vi "log_loop.vi"(8 "error in (no error)":errorcluster, 10 "Log queue":refnum<queue>, 11 "Message Queues":T4) -> (0 "error out":errorcluster)   [LabVIEW 2013]
doc: "Message loop for handling messages pertaining to the acquisition of data from the hardware."
uses:
  queues/que_all_message_queues.ctl
  queues/que_message_cluster.ctl
  gui/type_def/general_and_device.ctl
  gui/type_def/general.ctl
  gui/type_def/device.ctl
  log_state.ctl
  queues/que_enqueue_message_single.vi
  <vilib>/Utility/error.llb/Error Cluster From Error Code.vi
  <vilib>/ErrorRing/Error Ring.xnode
panel:
  out "gral_&_device":T1={"general"={"file_ext"="0.0.0.0", "TCP port"=0, "#devices"=0, "log?"=FALSE, "tcp?"=FALSE, "language"="ENG"}, "eeg_device"={"name"="", "hardware"="", "image"="", "path"=path "", "extra"="", "channels"=""}}
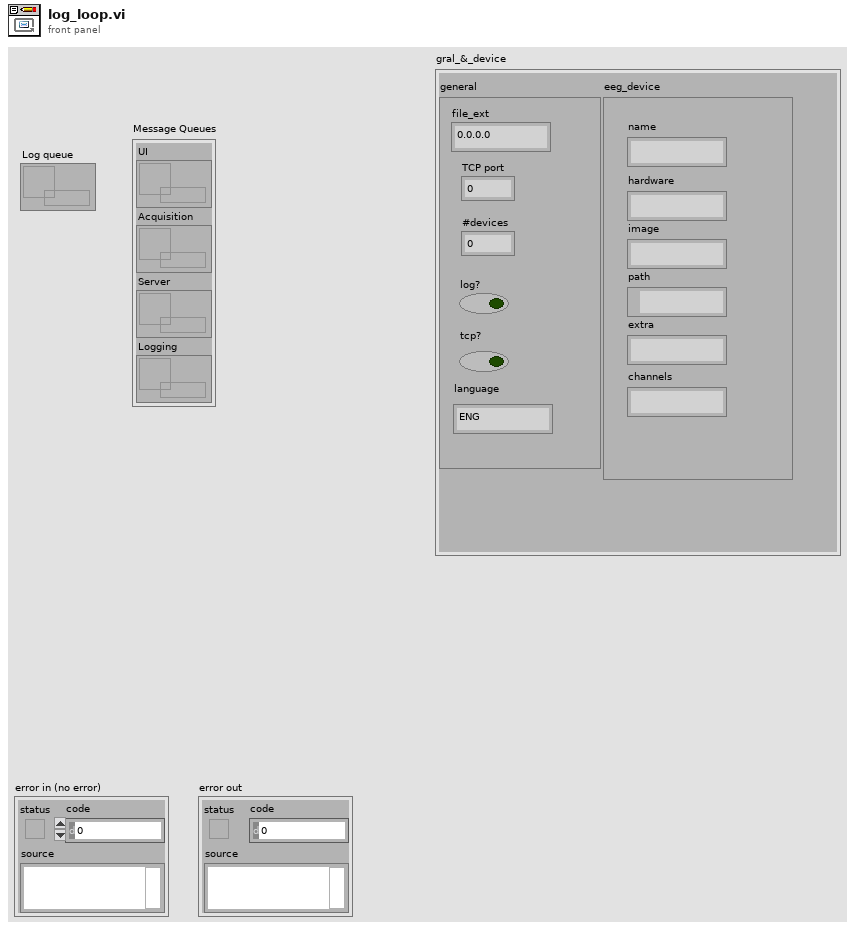
[diagram p1: front panel]
types:
  T1 = typedef "general_and_device.ctl" = cluster{"general":T2, "eeg_device":T3}
  T2 = typedef "general.ctl" = cluster{"file_ext":string, "TCP port":i32, "#devices":i32, "log?":bool, "tcp?":bool, "language":string}
  T3 = typedef "device.ctl" = cluster{"name":string, "hardware":string, "image":string, "path":path, "extra":string, "channels":string}
  T4 = typedef "que_all_message_queues.ctl" = cluster{"UI":refnum<queue>, "Acquisition":refnum<queue>, "Server":refnum<queue>, "Logging":refnum<queue>}
  T5 = typedef "log_state.ctl" = enum16{"Idle", "Logging"}
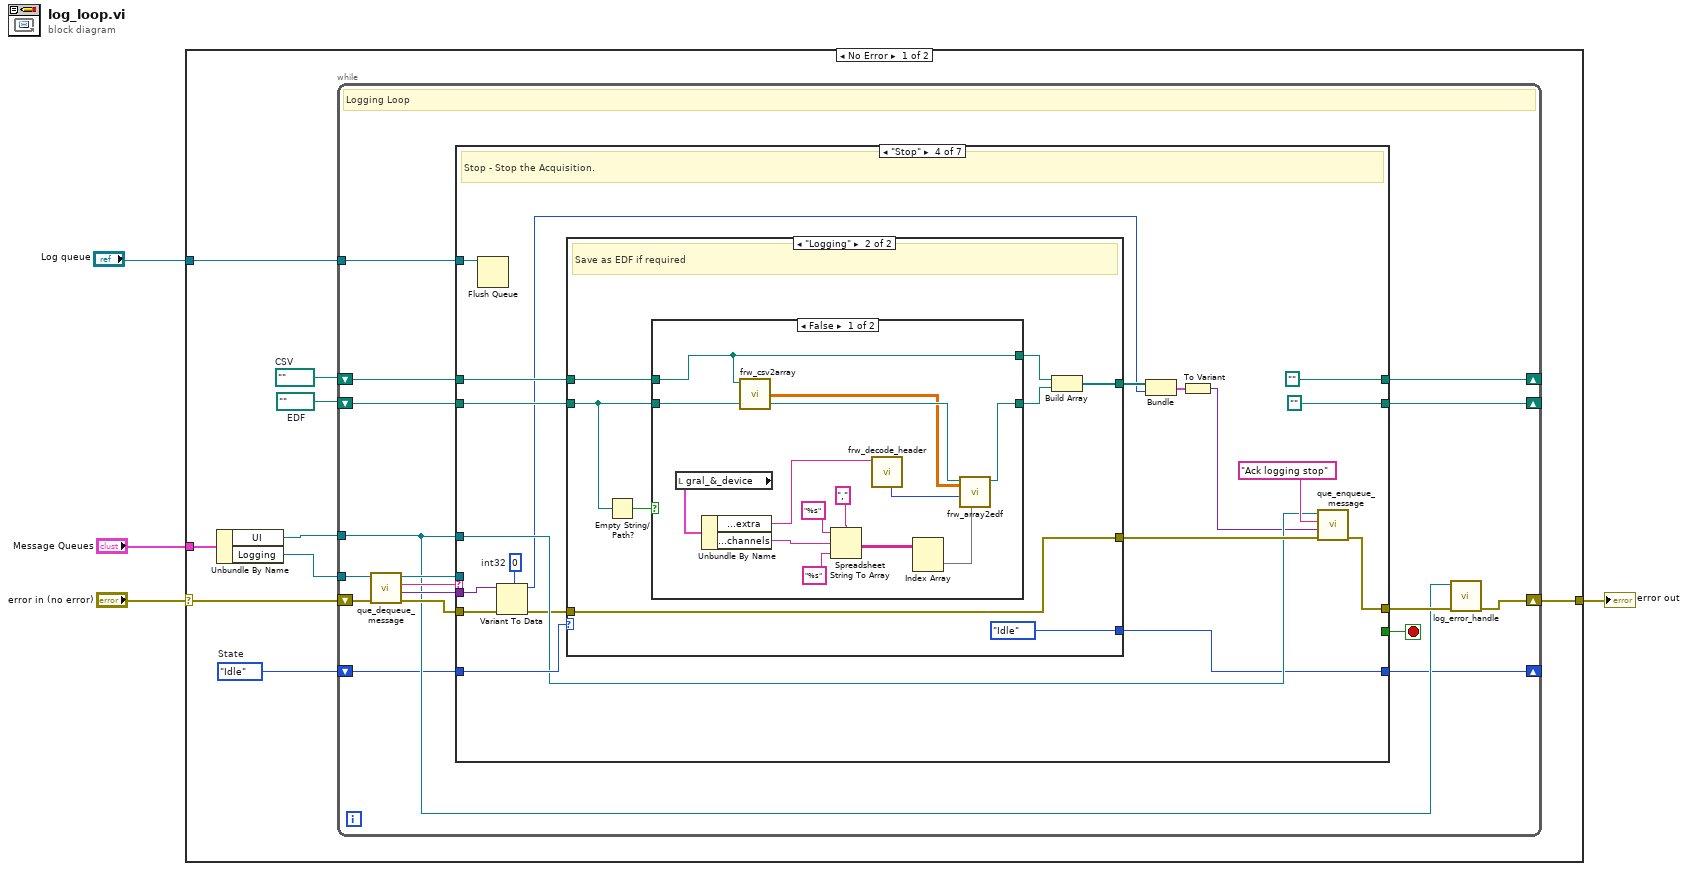
[diagram p0: block diagram]
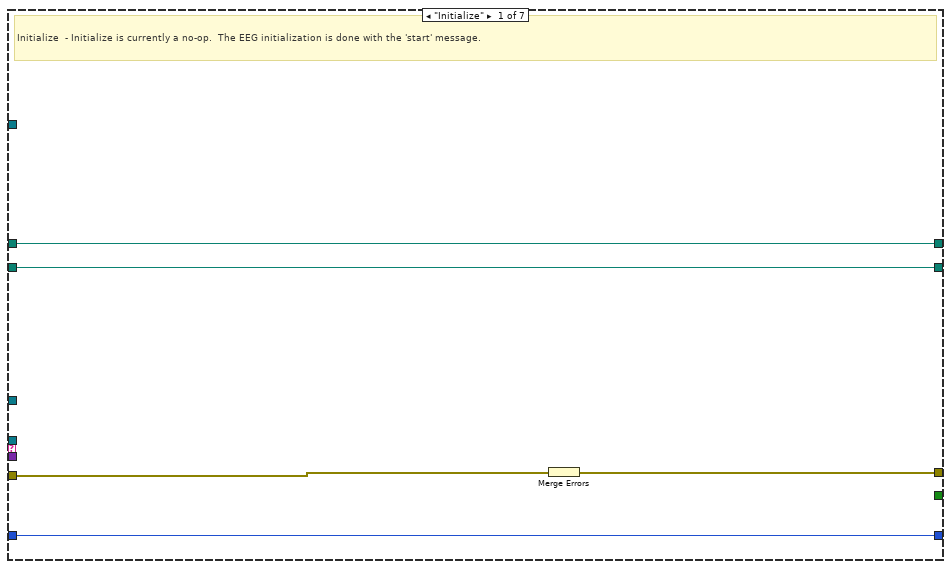
[diagram p2: hidden frame]
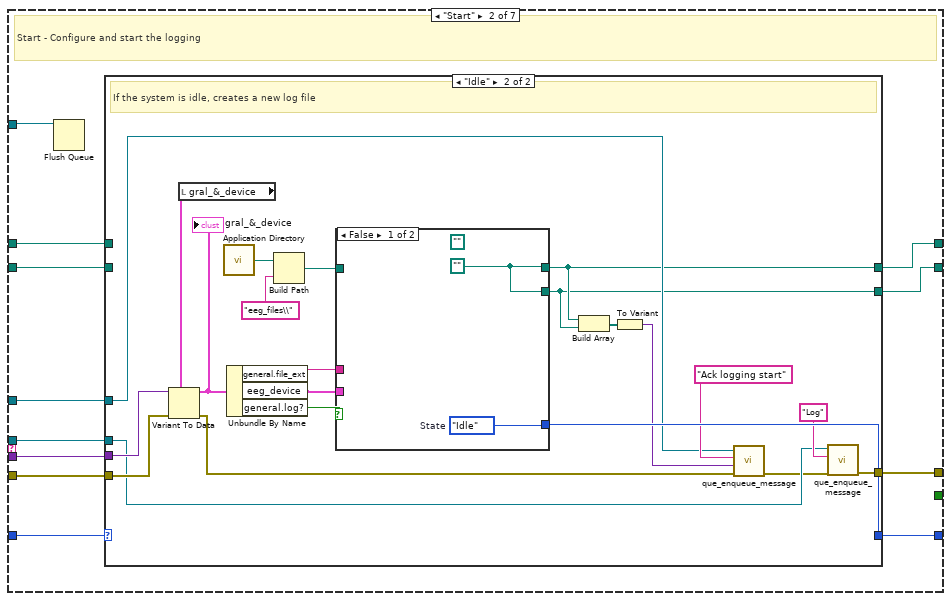
[diagram p3: hidden frame]
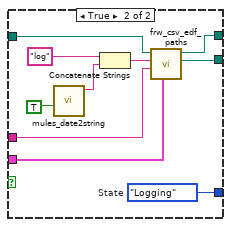
[diagram p5: hidden frame]
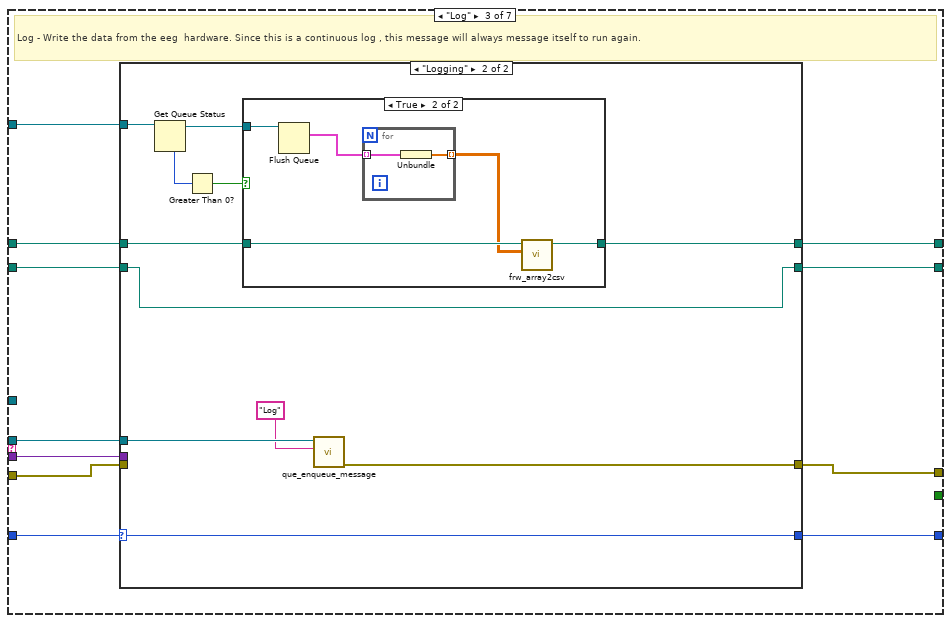
[diagram p6: hidden frame]
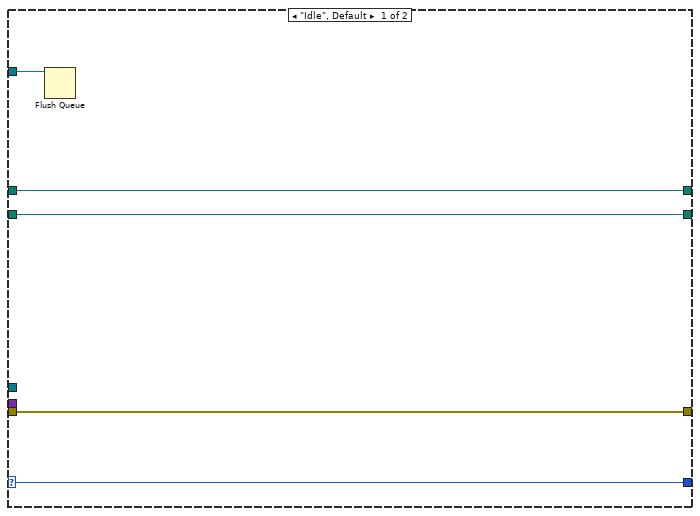
[diagram p7: hidden frame]
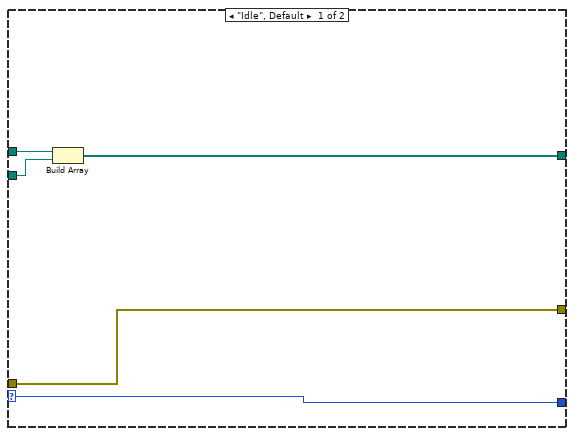
[diagram p9: hidden frame]
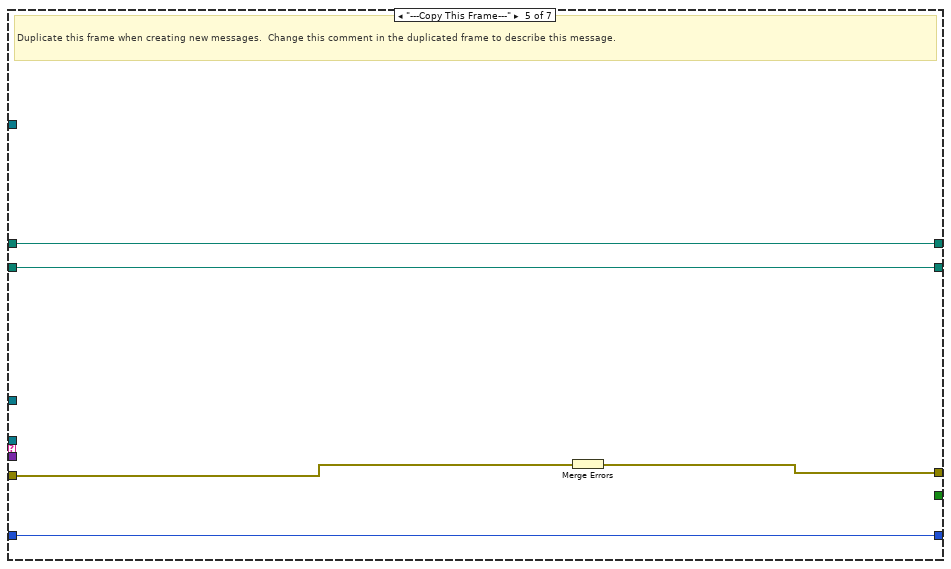
[diagram p11: hidden frame]
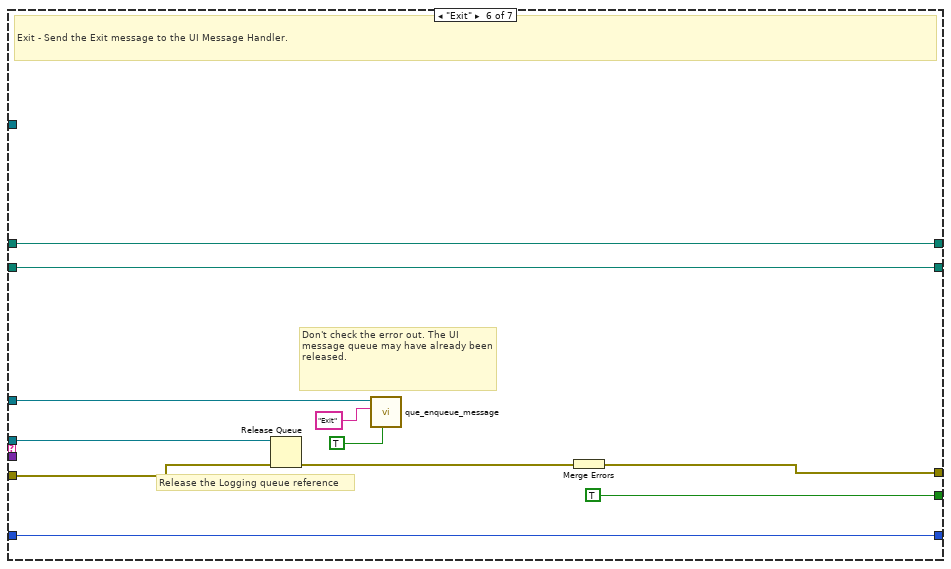
[diagram p12: hidden frame]
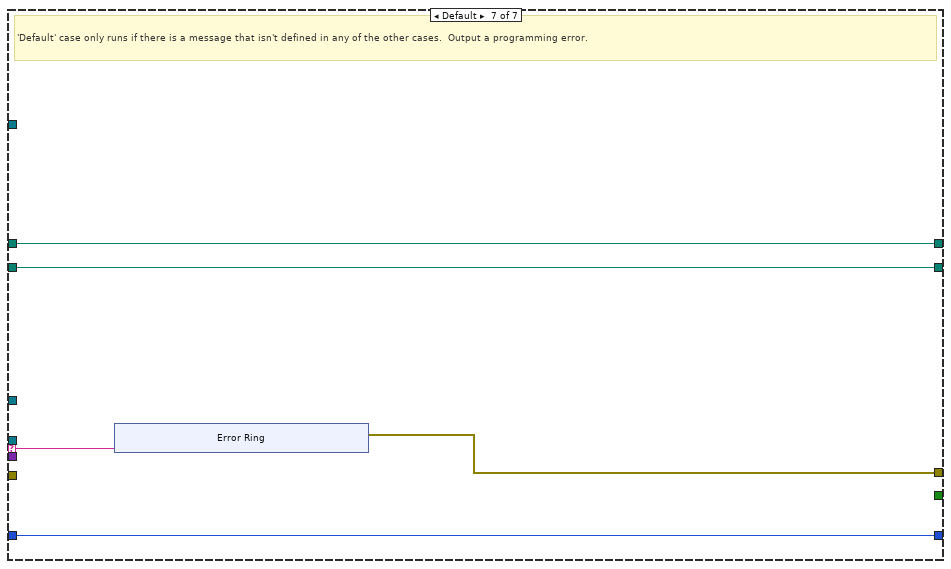
[diagram p13: hidden frame]
diagram:
  n1 = case shown="No Error" "error in (no error)" {
    selector: "error in (no error)" -> [w10 w196]
    tunnel: "Message Queues" -> [w13 _]
    tunnel: [w11 w196] -> w3
    tunnel: "Log queue" -> [w8 _]
    frame No Error {
      w5 = path ""  # EDF
      w7 = path ""  # CSV
      w6 = log_state."Idle"  # State
      n2 = Unbundle By Name(w13) -> ("UI"=w9:refnum<queue>, "Logging"=w12:refnum<queue>)
      n3 = while {
        tunnel: w12 -> [w25]
        shift-right: [w24] -> w11
        shift-left: w10 -> [w29]
        tunnel: w9 -> [w21]
        shift-right: [w20] -> _
        shift-left: w7 -> [w19]
        tunnel: w8 -> [w18]
        shift-right: [w16] -> _
        shift-left: w6 -> [w17]
        shift-right: [w14] -> _
        shift-left: w5 -> [w15]
        stop <- w30 stop-if-true
        # "Logging Loop"
        n4 = call "que_dequeue_message.vi"("error in (no error)"=w29, "Message Queue"=w25) -> ("error out"=w28:errorcluster, "Message Data"=w26:variant, "Message"=w27:string, "dup Message Queue"=w22:refnum<queue>)  [unwired: 6 in]
        n5 = case "Message Cases" shown="\"Stop\"" w27 {
          selector: w27 -> [_ _ _ _ _ _ w186]
          tunnel: w22 -> [_ w47 w95 _ _ w176 _]
          tunnel: w28 -> [w34 w40 w94 w127 w172 w180 _]
          tunnel: [w35 w37 w96 w133 w171 w182 w187] -> w23
          tunnel: [_ _ _ _ _ TRUE _] -> w30
          tunnel: w26 -> [_ w44 w91 w126 _ _ _]
          tunnel: w21 -> [_ w41 _ w135 _ w181 _]
          tunnel: w17 -> [w33 w45 w92 w138 w170 w175 w188]
          tunnel: [w33 w46 w93 w134 w170 w175 w188] -> w16
          tunnel: [w32 w43 w87 path "" w169 w174 w185] -> w20
          tunnel: w19 -> [w32 w42 w90 w137 w169 w174 w185]
          tunnel: w18 -> [_ w36 w89 w121 _ _ _]
          tunnel: w15 -> [w31 w39 w88 w130 w168 w173 w184]
          tunnel: [w31 w38 w86 path "" w168 w173 w184] -> w14
          frame "Initialize" {
            # "Initialize  - Initialize is currently a no-op.  The EEG initialization is done with the 'start' message."
            n6 = Merge Errors(w34) -> (w35:errorcluster)
          }
          frame "Start" {
            # "Start - Configure and start the logging"
            n7 = Flush Queue(queue=w36) -> ()  [unwired: 1 in, 3 out]
            n8 = case shown="\"Idle\"" w45 {
              selector: w45 -> [w50 _]
              tunnel: [w51 w64] -> w37
              tunnel: w40 -> [w51 w72]
              tunnel: w47 -> [_ w60]
              tunnel: [w50 w66] -> w46
              tunnel: w44 -> [_ w73]
              tunnel: [w49 w55] -> w43
              tunnel: w42 -> [w49 _]
              tunnel: w41 -> [_ w57]
              tunnel: w39 -> [w48 _]
              tunnel: [w48 w54] -> w38
              frame "Logging" {
                # "The system is already acquiring. Ignore the \"Start\" message."
              }
              frame "Idle" {
                # "If the system is idle, creates a new log file"
                n9 = local read "gral_&_device"() -> (w71:T1)
                n10 = Variant To Data(error in=w72, type=w71, Variant=w73) -> (data=w70:T1, error out=w56:errorcluster)
                "gral_&_device" <- w70
                n11 = call <vilib>:"Application Directory.vi"() -> ("Application Directory"=w62:path)
                n12 = Unbundle By Name(w70) -> ("general.file_ext"=w67:string, "eeg_device"=w68:T3, "general.log?"=w69:bool)
                n13 = Build Path(base path=w62, name or relative path="eeg_files\\") -> (appended path=w61:path)
                n14 = case shown="False" w69 {
                  tunnel: w68 -> [_ w83]
                  tunnel: w67 -> [_ w85]
                  tunnel: [w74 w79] -> w55
                  tunnel: [w74 w78] -> w54
                  tunnel: [w75 w77] -> w66
                  tunnel: w61 -> [_ w76]
                  frame False {
                    w75 = log_state."Idle"  # State
                    w74 = path ""
                    (unwired) path ""
                  }
                  frame True {
                    w77 = log_state."Logging"  # State
                    n15 = call "mules_date2string.vi"("seconds?"=TRUE) -> ("date_time_string"=w81:string)  [unwired: 8 in, 2 out]
                    n16 = Concatenate Strings("log" ("string"), w81) -> (w80:string)
                    n17 = call "frw_csv_edf_paths.vi"("eeg_device"=w83, "file_extension"=w85, "filename"=w80, "directory path"=w76) -> ("path edf"=w78:path, "path csv"=w79:path)  [unwired: 6 in]
                  }
                }
                n18 = Build Array(w55, w54) -> (w53:path[])
                n19 = To Variant(anything=w53) -> (Variant=w52:variant)
                n20 = call-poly "que_enqueue_message.vi"("error in (no error)"=w56, "Message Data"=w52, "Message"="Ack logging start", "Message Queue"=w57) -> ("error out"=w58:errorcluster)  [unwired: 6 in, 1 out]
                n21 = call-poly "que_enqueue_message.vi"("error in (no error)"=w58, "Message"="Log", "Message Queue"=w60) -> ("error out"=w64:errorcluster)  [unwired: 7 in, 1 out]
              }
            }
          }
          frame "Log" {
            # "Log - Write the data from the eeg  hardware. Since this is a continuous log , this message will always message itself to run again."
            n22 = case shown="\"Logging\"" w92 {
              selector: w92 -> [w100 w112]
              tunnel: [w101 w111] -> w96
              tunnel: w95 -> [_ w110]
              tunnel: w94 -> [w101 _]
              tunnel: [w100 w112] -> w93
              tunnel: w91 -> [_ _]
              tunnel: w90 -> [w99 w109]
              tunnel: w89 -> [w97 w104]
              tunnel: w88 -> [w98 w106]
              tunnel: [w99 w108] -> w87
              tunnel: [w98 w106] -> w86
              frame "Idle", Default {
                # "Ignore \"Acquire\" messages when the acquisition is idle."
                n23 = Flush Queue(queue=w97) -> ()  [unwired: 1 in, 3 out]
              }
              frame "Logging" {
                # "Acquire more data while in the \"Acquiring\" state."
                n24 = Get Queue Status(queue=w104) -> (queue out=w102:refnum<queue>, # elements in queue=w103:i32)  [unwired: 2 in, 6 out]
                n25 = Greater Than 0?(x=w103) -> (x > 0?=w105:bool)
                n26 = case shown="True" w105 {
                  tunnel: w109 -> [w113 w118]
                  tunnel: [w113 w117] -> w108
                  tunnel: w102 -> [_ w115]
                  frame False {
                  }
                  frame True {
                    n27 = Flush Queue(queue=w115) -> (remaining elements=w114:cluster{dbl[]}[])  [unwired: 1 in, 2 out]
                    n28 = for {
                      tunnel: w114 -> [w120] mode=indexing
                      tunnel: [w119] -> w116 mode=indexing
                      n29 = Unbundle(w120) -> (w119:dbl[])
                    }
                    n30 = call "frw_array2csv.vi"("2Darray"=w116, "file path in"=w118) -> ("path out"=w117:path)  [unwired: 8 in, 1 out]
                  }
                }
                n31 = call-poly "que_enqueue_message.vi"("Message"="Log", "Message Queue"=w110) -> ("error out"=w111:errorcluster)  [unwired: 8 in, 1 out]
              }
            }
          }
          frame "Stop" {
            w128 = 0  # int32
            # "Stop - Stop the Acquisition."
            n32 = Flush Queue(queue=w121) -> ()  [unwired: 1 in, 3 out]
            n33 = Variant To Data(error in=w127, type=w128, Variant=w126) -> (data=w125:i32, error out=w122:errorcluster)
            n34 = case shown="\"Logging\"" w138 {
              selector: w138 -> [w144 _]
              tunnel: [w143 w151] -> w136
              tunnel: w137 -> [w142 w146]
              tunnel: w122 -> [w143 w151]
              tunnel: [w144 log_state."Idle" ("State")] -> w134
              tunnel: w130 -> [w141 w150]
              tunnel: [w140 w145] -> w129
              frame "Idle", Default {
                n35 = Build Array(w142, w141) -> (w140:path[])
              }
              frame "Logging" {
                # "Save as EDF if required"
                n36 = Empty String/Path?(string/path=w150) -> (empty?=w149:bool)
                n37 = case shown="False" w149 {
                  tunnel: w150 -> [w156 w166]
                  tunnel: [w153 w166] -> w148
                  tunnel: [w155 w167] -> w147
                  tunnel: w146 -> [w155 w167]
                  frame False {
                    n38 = local read "gral_&_device"() -> (w165:T1)
                    n39 = Unbundle By Name(w165) -> ("eeg_device.extra"=w164:string, "eeg_device.channels"=w161:string)
                    n40 = call "frw_csv2array.vi"("file path"=w155) -> ("values"=w154:dbl[][])  [unwired: 7 in, 3 out]
                    n41 = Spreadsheet String To Array(delimiter (Tab)=",", format string="%s" ("delimiter (Tab)"), spreadsheet string=w161, array type (2D Dbl)="%s" ("delimiter (Tab)")) -> (array=w158:string[][])
                    n42 = call "frw_decode_header.vi"("header1"=w164) -> ("fs"=w163:i32)  [unwired: 5 in, 5 out]
                    n43 = Index Array(array=w158) -> (element=w157:string[])  [unwired: 2 in]
                    n44 = call "frw_array2edf.vi"("channel names"=w157, "fs"=w163, "2D array"=w154, "file path"=w156) -> ("path out"=w153:path)  [unwired: 6 in, 1 out]
                  }
                  frame True {
                  }
                }
                n45 = Build Array(w147, w148) -> (w145:path[])
              }
            }
            n46 = Bundle(w129, "int32"=w125) -> (w124:cluster{path[], "int32":i32})  [unwired: 1 in]
            n47 = To Variant(anything=w124) -> (Variant=w123:variant)
            n48 = call-poly "que_enqueue_message.vi"("error in (no error)"=w136, "Message Data"=w123, "Message"="Ack logging stop", "Message Queue"=w135) -> ("error out"=w133:errorcluster)  [unwired: 6 in, 1 out]
          }
          frame "---Copy This Frame---" {
            # "Duplicate this frame when creating new messages.  Change this comment in the duplicated frame to describe this message."
            n49 = Merge Errors(w172) -> (w171:errorcluster)
          }
          frame "Exit" {
            # "Don't check the error out. The UI message queue may have already been released."
            # "Release the Logging queue reference"
            # "Exit - Send the Exit message to the UI Message Handler."
            n50 = Release Queue(queue=w176, error in (no error)=w180) -> (error out=w177:errorcluster)  [unwired: 1 in, 2 out]
            n51 = call-poly "que_enqueue_message.vi"("Priority Message? (F)"=TRUE, "Message"="Exit", "Message Queue"=w181) -> ()  [unwired: 7 in, 2 out]
            n52 = Merge Errors(w177) -> (w182:errorcluster)
          }
          frame Default {
            # "'Default' case only runs if there is a message that isn't defined in any of the other cases.  Output a programming error."
            n53 = xnode "Error Ring"("parameter 0"=w186) -> ("error out"=w187:errorcluster)
          }
        }
        n54 = call "log_error_handle.vi"("error in (no error)"=w23, "Message Queue"=w21) -> ("dup error in"=w24:errorcluster)  [unwired: 8 in, 1 out]
      }
    }
    frame Error {
    }
  }
  "error out" <- w3
